vi "Read Exception Status.vi"(7 "unit ID":u8, 8 "error in":errorcluster, 11 "Modbus master in":refnum<class "Modbus Master.lvclass">) -> (0 "error out":errorcluster, 2 "exception status":u8, 3 "Modbus master out":refnum<class "Modbus Master.lvclass">)   [LabVIEW 2013, in "Modbus Library - Advance.lvlib" / "Modbus Master.lvclass"]
doc: "Interface to reads any exception status set in the device. The exeption status is a set of 8 status bits, packed as a U8 integer. With third-party devices, this function should only be used if the device is a serial device, as the Modbus specification defines this as a serial-only function. However, this library includes support for this function regardless of the transport mechanism."
uses:
  Modbus Master.lvclass
  Modbus API.lvclass/Modbus API.ctl
  Transmission Data Unit/Serial Interface/Serial Data Unit.lvclass
  Modbus Master.lvclass/Modbus Master.ctl
  Transmission Data Unit/Transmission Data Unit.lvclass/Transmission Data Unit.ctl
  Transmission Data Unit/Transmission Data Unit.lvclass
  Modbus API.lvclass
  Master Function Definition/Master Function Definition.lvclass
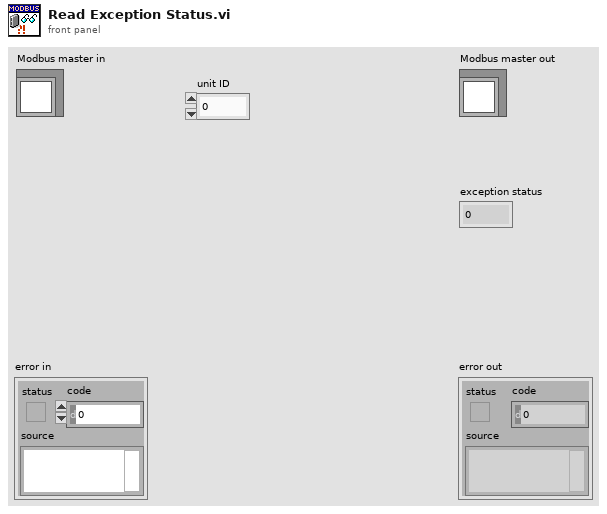
[diagram p1: front panel]
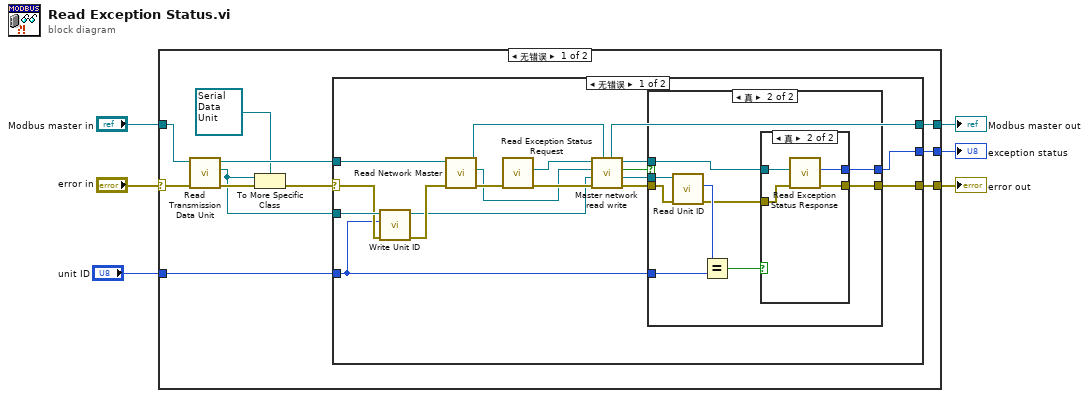
[diagram p0: block diagram]
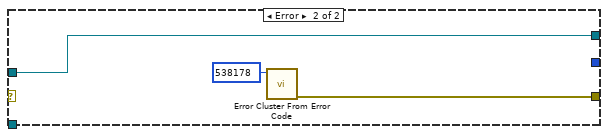
[diagram p4: hidden frame]
diagram:
  n1 = case shown="无错误" "error in" {
    selector: "error in" -> [w12 w54]
    tunnel: [w16 w55] -> w6
    tunnel: "Modbus master in" -> [w15 w55]
    tunnel: [w14 _] -> w4
    tunnel: [w13 w54] -> w3
    tunnel: "unit ID" -> [w7 _]
    frame No Error {
      n2 = call "Read Transmission Data Unit.vi"("error in"=w12, "Modbus instance in"=w15) -> ("error out"=w11:errorcluster, "transmission data unit"=w10:refnum<class "Transmission Data Unit.lvclass">, "Modbus instance out"=w17:refnum<class "Modbus Master.lvclass">)  [unwired: 7 in]
      n3 = To More Specific Class(target class=refnum<class "Serial Data Unit.lvclass"> refnum ("Serial Data Unit"), reference=w10, error in=w11) -> (error out=w8:errorcluster)  [unwired: 1 out]
      n4 = case shown="无错误" w8 {
        selector: w8 -> [w22 _]
        tunnel: w17 -> [w35 w52]
        tunnel: [w30 w52] -> w16
        tunnel: [w28 _] -> w14
        tunnel: [w25 w53] -> w13
        tunnel: w10 -> [w23 _]
        tunnel: w7 -> [w18 _]
        frame No Error {
          n5 = call "Write Unit ID.vi"("error in"=w22, "unit ID"=w18, "transmission data unit in"=w23) -> ("error out"=w21:errorcluster, "transmission data unit out"=w20:refnum<class "Transmission Data Unit.lvclass">)  [unwired: 7 in]
          n6 = call "Read Network Master.vi"("error in"=w21, "Modbus master in"=w35) -> ("error out"=w32:errorcluster, "network master"=w29:refnum<class "Network Master.lvclass">, "Modbus master out"=w31:refnum<class "Modbus Master.lvclass">)  [unwired: 7 in]
          n7 = call "Read Exception Status Request.vi"("error in"=w32) -> ("error out"=w34:errorcluster, "modbus data unit out"=w33:refnum<class "Modbus Data Unit.lvclass">)  [unwired: 9 in]
          n8 = call "Master network read write.vi"("Modbus master in"=w31, "error in"=w34, "transmission data unit in"=w20, "network master in"=w29, "Modbus data unit in"=w33) -> ("error out"=w26:errorcluster, "transmission data unit out"=w19:refnum<class "Transmission Data Unit.lvclass">, "PDU Valid?"=w24:bool, "Modbus data unit out"=w27:refnum<class "Modbus Data Unit.lvclass">, "Modbus master out"=w30:refnum<class "Modbus Master.lvclass">)  [unwired: 2 in]
          n9 = case shown="真" w24 {
            tunnel: [_ w45] -> w28
            tunnel: w27 -> [_ w44]
            tunnel: w26 -> [w36 w41]
            tunnel: [w36 w43] -> w25
            tunnel: w19 -> [_ w42]
            tunnel: w18 -> [_ w39]
            frame False {
            }
            frame True {
              n10 = call "Read Unit ID.vi"("error in"=w41, "transmission data unit in"=w42) -> ("error out"=w37:errorcluster, "unit ID"=w40:u8)  [unwired: 7 in, 1 out]
              n11 = Equal?(x=w40, y=w39) -> (x = y?=w38:bool)
              n12 = case shown="真" w38 {
                tunnel: [_ w50] -> w45
                tunnel: w44 -> [_ w49]
                tunnel: [w46 w48] -> w43
                tunnel: w37 -> [w46 w47]
                frame False {
                }
                frame True {
                  n13 = call "Read Exception Status Response.vi"("error in"=w47, "modbus data unit in"=w49) -> ("error out"=w48:errorcluster, "Exception Status"=w50:u8)  [unwired: 8 in]
                }
              }
            }
          }
        }
        frame Error {
          n14 = call <vilib>:"Error Cluster From Error Code.vi"("error code (0)"=538178) -> ("error out"=w53:errorcluster)  [unwired: 8 in]
        }
      }
    }
    frame Error {
    }
  }
  "error out" <- w3
  "Modbus master out" <- w6
  "exception status" <- w4
